vi "cores_global_ECO.vi"() -> (0 "LVutils global ECO":i32=19940000)   [LabVIEW 2015]
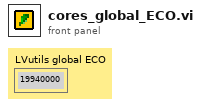
[diagram p1: front panel]
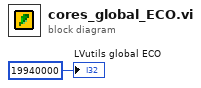
[diagram p0: block diagram]
diagram:
  "LVutils global ECO" <- 19940000
